vi "test_tcpbuf.vi"() -> ()   [LabVIEW 2017]
panel:
  in  "stop":bool
  in  "use":bool
  in  "add":bool
  out "element 2":string
  out "element":string
  in  "exit":bool
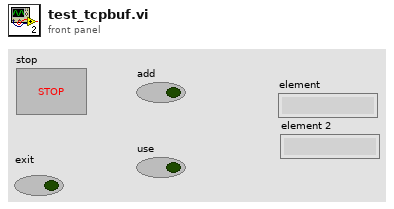
[diagram p1: front panel]
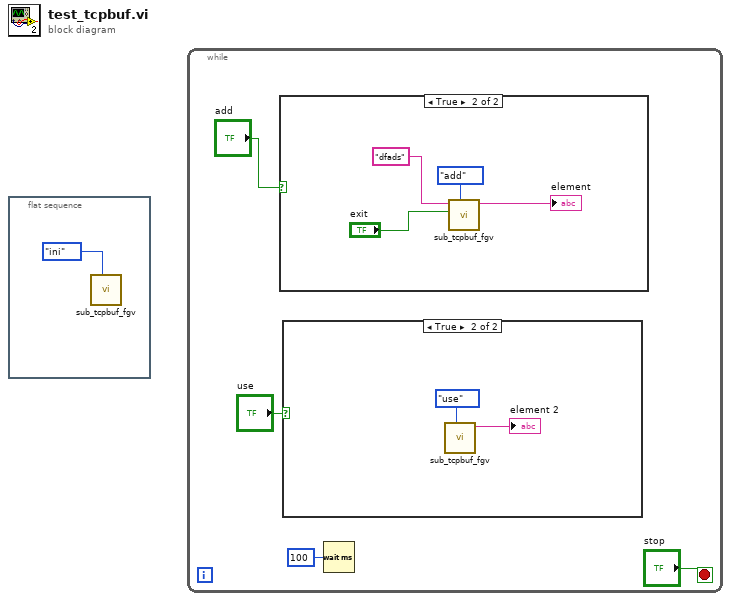
[diagram p0: block diagram]
diagram:
  n1 = flat-sequence {
    frame #0 {
      n2 = call "sub_tcpbuf_fgv.vi"("cmd"=enum16{"ini", "add", "use"}."ini") -> ()  [unwired: 8 in, 3 out]
    }
  }
  n3 = while {
    stop <- "stop" stop-if-true
    n4 = case shown="True" "add" {
      frame False {
      }
      frame True {
        n5 = call "sub_tcpbuf_fgv.vi"("cmd"=enum16{"ini", "add", "use", "check"}."add", "exit"="exit", "cmd_str"="dfads") -> ("element"=→"element":string)  [unwired: 6 in, 2 out]
      }
    }
    n6 = case shown="True" "use" {
      frame False {
      }
      frame True {
        n7 = call "sub_tcpbuf_fgv.vi"("cmd"=enum16{"ini", "add", "use", "check"}."use") -> ("element"=→"element 2":string)  [unwired: 8 in, 2 out]
      }
    }
    n8 = Wait (ms)(milliseconds to wait=u32 100) -> ()  [unwired: 1 out]
  }
